vi "Sensor Range Control.vi"() -> ()   [LabVIEW 2013]
uses:
  <vilib>/myRIO/Instrument Drivers/Onboard IO/DIO/vis/Smart Open.vi
  <vilib>/myRIO/Instrument Drivers/Onboard IO/DIO/vis/Write.vi
  <vilib>/myRIO/Instrument Drivers/Onboard IO/DIO/vis/Read.vi
  <vilib>/myRIO/Instrument Drivers/Onboard IO/DIO/vis/Open.vi
  <vilib>/myRIO/Common/Instrument Driver Framework/myRIO v1.0/DIO/vis/myRIO v1.1 Open DIO.vi
  <vilib>/myRIO/Common/Instrument Driver Framework/Utilities/vis/Validate Channels.vi
  <vilib>/myRIO/Common/Instrument Driver Framework/myRIO v1.0/DIO/vis/myRIO v1.0 Reserve DIO.vi
  <vilib>/myRIO/Common/Instrument Driver Framework/myRIO v1.0/Resource Manager/vis/myRIO v1.0 Reserve Channel List.vi
  <vilib>/myRIO/Common/Instrument Driver Framework/myRIO v1.0/DIO/vis/myRIO v1.0 Build MUX Configuration DIO.vi
  <vilib>/myRIO/Common/Instrument Driver Framework/myRIO v1.0/Resource Manager/vis/myRIO v1.0 Reserve Channel.vi
  <vilib>/myRIO/Common/Instrument Driver Framework/myRIO v1.0/Resource Manager/vis/myRIO v1.0 Unreserve Channel.vi
  <vilib>/myRIO/Common/Instrument Driver Framework/myRIO v1.0/Resource Manager/vis/myRIO v1.0 Create Configuration List.vi
  <vilib>/myRIO/Common/Instrument Driver Framework/myRIO v1.0/Resource Manager/vis/myRIO v1.0 Build Mutex Name.vi
  <vilib>/myRIO/Common/Instrument Driver Framework/myRIO v1.0/myRIO v1.1 Open.vi
  <vilib>/Utility/VariantDataType/GetNumericInfo.vi
  <vilib>/Utility/error.llb/Error Cluster From Error Code.vi
  <vilib>/myRIO/Common/Instrument Driver Framework/Utilities/vis/IO Manager.vi
  <vilib>/myRIO/Common/Instrument Driver Framework/Utilities/vis/Configuration Manager.vi
  <vilib>/myRIO/Common/Instrument Driver Framework/myRIO v1.0/Resource Manager/vis/myRIO v1.0 Configure IO.vi
  <vilib>/myRIO/Common/Instrument Driver Framework/myRIO v1.0/myRIO v1.0 Close.vi
  <vilib>/myRIO/Common/Instrument Driver Framework/myRIO v1.0/DIO/vis/myRIO v1.0 Write DIO.vi
  <vilib>/myRIO/Common/Instrument Driver Framework/myRIO v1.0/DIO/vis/myRIO v1.0 Read DIO.vi
panel:
  out "Distance (m)":dbl
  in  "Stop":bool=TRUE
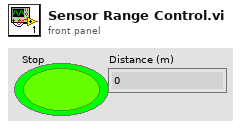
[diagram p1: front panel]
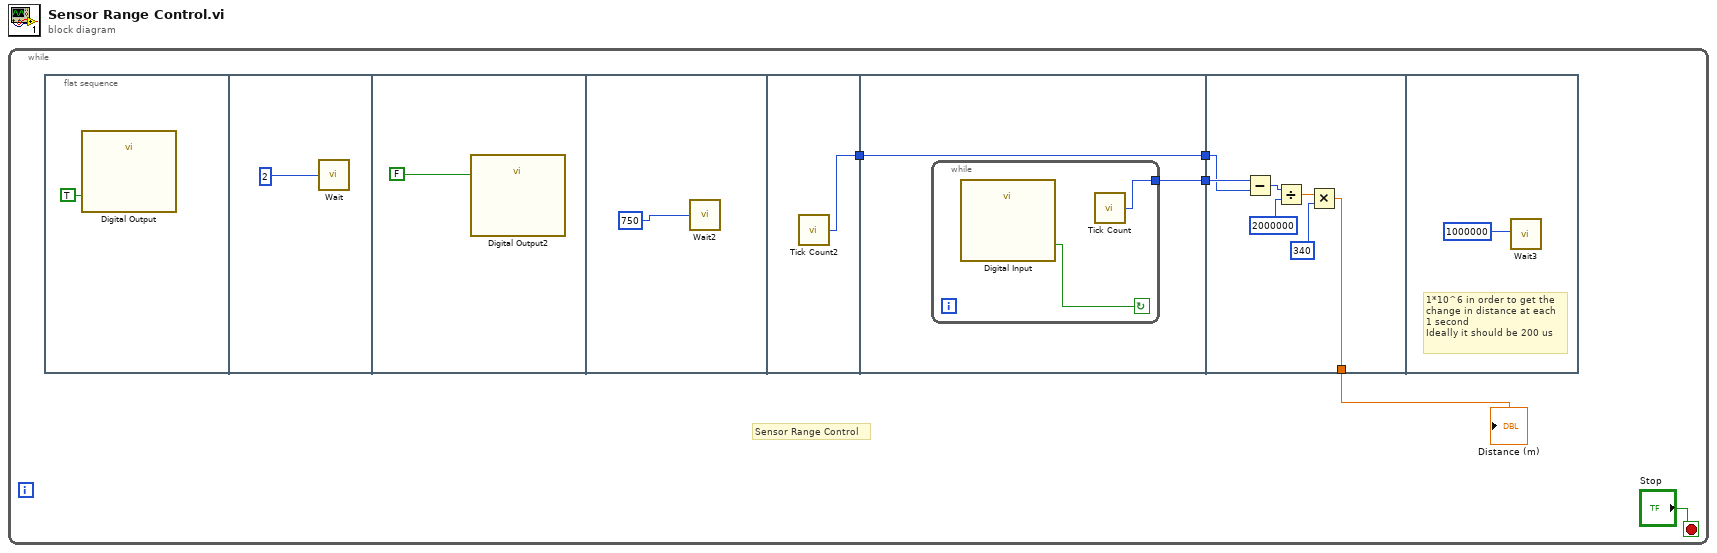
[diagram p0: block diagram]
diagram:
  n1 = while {
    stop <- "Stop" stop-if-true
    # "Sensor Range Control"
    n2 = flat-sequence {
      tunnel: [w10] -> w2
      tunnel: [w12] -> w4
      tunnel: [w11] -> w3
      tunnel: w2 -> [w11]
      tunnel: w4 -> [w21]
      tunnel: w3 -> [w16]
      tunnel: [w15] -> w1
      frame #0 {
        n3 = call "Digital Output"("A/DIO0 (Pin 11)"=TRUE ("C/DIO7")) -> ()  [unwired: 26 in, 1 out]
      }
      frame #1 {
        n4 = call "Wait"("Count(uSec)"=2) -> ()  [unwired: 1 out]
      }
      frame #2 {
        n5 = call "Digital Output2"("A/DIO0 (Pin 11)"=FALSE ("Boolean")) -> ()  [unwired: 26 in, 1 out]
      }
      frame #3 {
        n6 = call "Wait2"("Count(uSec)"=750) -> ()  [unwired: 1 out]
      }
      frame #4 {
        n7 = call "Tick Count2"() -> ("Tick Count(uSec)"=w10:u32)
      }
      frame #5 {
        n8 = while {
          tunnel: [w13] -> w12
          stop <- w14 continue-if-true
          n9 = call "Digital Input"() -> ("A/DIO0 (Pin 11)"=w14:bool)  [unwired: 26 in, 1 out]
          n10 = call "Tick Count"() -> ("Tick Count(uSec)"=w13:u32)
        }
      }
      frame #6 {
        n11 = Subtract(x=w21, y=w16) -> (x-y=w20:u32)
        n12 = Divide(x=w20, y=2000000) -> (x/y=w18:dbl)
        n13 = Multiply(x=w18, y=340) -> (x*y=w15:dbl)
      }
      frame #7 {
        # "1*10^6 in order to get the\nchange in distance at each\n1 second\nIdeally it should be 200 us"
        n14 = call "Wait3"("Count(uSec)"=1000000) -> ()  [unwired: 1 out]
      }
    }
    "Distance (m)" <- w1
  }
